vi "Refresh Target List.vi"(6 "Supported Devices":u32[](array[numeric]), 8 "error in (no error)":errorcluster, 9 "OwningVI Ref":refnum<vi>, 10 "UI Ref Cluster":T4, 11 "Target Info Cache":T1={"USBTargetList"={"TargetList"=[], "Value"=-1, "Target RT Info List"=[]}, "WiFiTargetList"={"TargetList"=[], "Value"=-1, "Target RT Info List"=[]}, "GenericTargetList"={"TargetList"=[], "Value"=-1, "Target RT Info List"=[]}, "IPTargetList"={"IP Error Out"={"status"=FALSE, "code"=0, "source"=""}, "Target RT Info List"=[]}} {"IPTargetList"."Target RT Info List"."ProdID" format="%.0x"; "USBTargetList"."Target RT Info List"."ProdID" format="%.0x"; "WiFiTargetList"."Target RT Info List"."ProdID" format="%.0x"; "GenericTargetList"."Target RT Info List"."ProdID" format="%.0x"}) -> (0 "error out":errorcluster, 3 "Target Info Cache Output":T1 {"IPTargetList"."Target RT Info List"."ProdID" format="%.0x"; "USBTargetList"."Target RT Info List"."ProdID" format="%.0x"; "WiFiTargetList"."Target RT Info List"."ProdID" format="%.0x"; "GenericTargetList"."Target RT Info List"."ProdID" format="%.0x"})   [LabVIEW 2021, in "myRIOMetaDataObj.lvclass"]
uses:
  myRIOMetaDataObj.lvclass
  WizardUIRef.ctl
  AvailableTargets.ctl
  TargetInfoHistory.ctl
  TargetListInfo.ctl
  <resource>/myRIO/Target Info.ctl
  InternalErrorCodes.vi
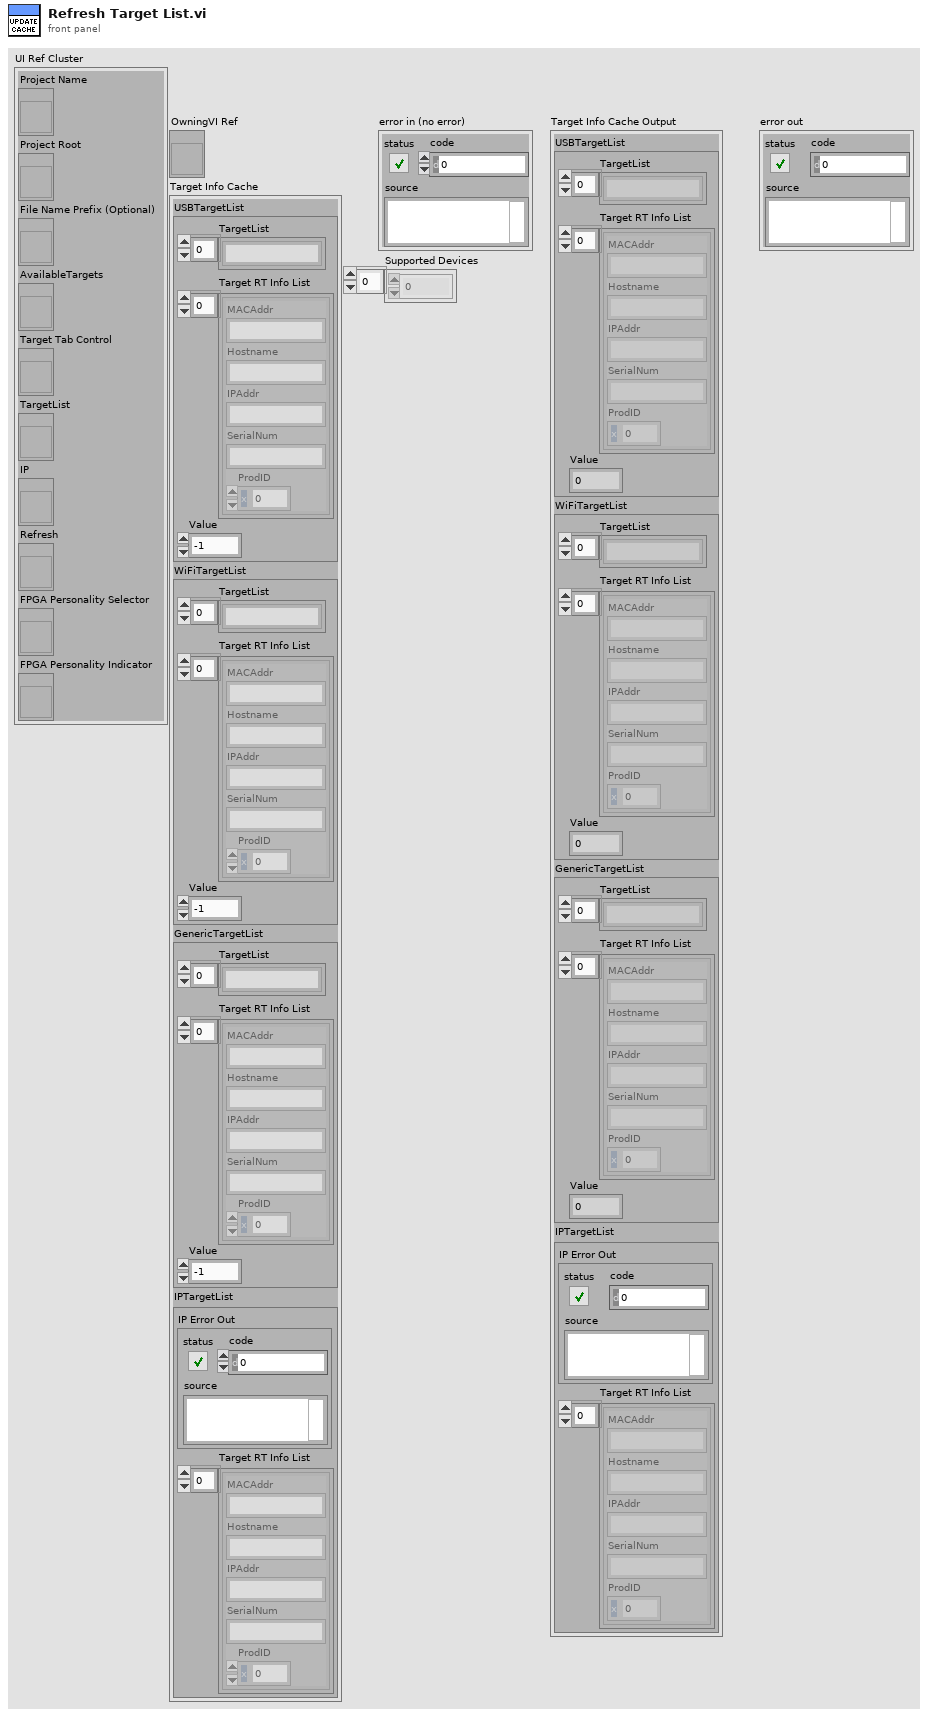
[diagram p1: front panel]
types:
  T1 = typedef "myRIOMetaDataObj.lvclass/TargetInfoHistory.ctl" = cluster{"USBTargetList":T2, "WiFiTargetList":T2, "GenericTargetList":T2, "IPTargetList":cluster{"IP Error Out":errorcluster, "Target RT Info List":T3[]}}
  T2 = typedef "myRIOMetaDataObj.lvclass/TargetListInfo.ctl" = cluster{"TargetList":string[], "Value":i32, "Target RT Info List":T3[]}
  T3 = typedef "Target Info.ctl" = cluster{"MACAddr":string, "Hostname":string, "IPAddr":string, "SerialNum":string, "ProdID":u32}
  T4 = typedef "myRIOMetaDataObj.lvclass/WizardUIRef.ctl" = cluster{"Project Name":refnum<vi>, "Project Root":refnum<vi>, "File Name Prefix (Optional)":refnum<vi>, "AvailableTargets":refnum<vi>, "Target Tab Control":refnum<vi>, "TargetList":refnum<vi>, "IP":refnum<vi>, "Refresh":refnum<vi>, "FPGA Personality Selector":refnum<vi>, "FPGA Personality Indicator":refnum<vi>}
  T5 = enum8{"Enabled", "Disabled", "Disabled and Grayed Out"}
  T6 = enum32{"USBTarget", "WifiTarget", "NoSpecificTarget", "TargetIP"}
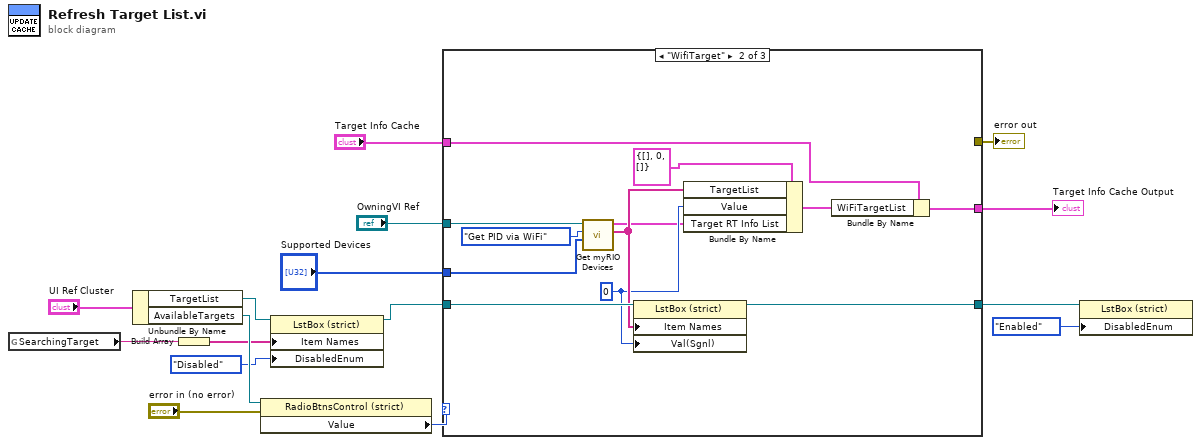
[diagram p0: block diagram]
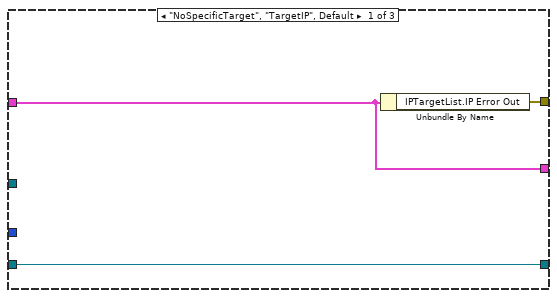
[diagram p2: hidden frame]
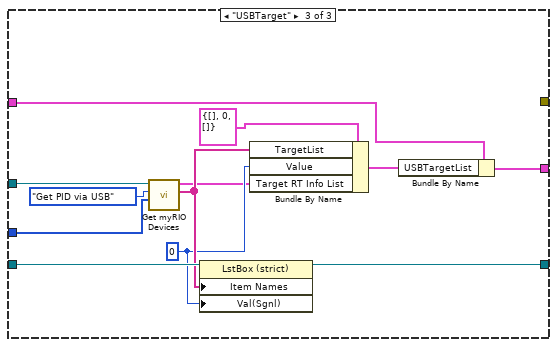
[diagram p3: hidden frame]
diagram:
  n1 = global read "InternalErrorCodes.vi" "SearchingTarget"() -> (w9:string)
  n2 = Unbundle By Name("UI Ref Cluster") -> ("TargetList"=w11:refnum<vi>, "AvailableTargets"=w15:refnum<vi>)
  n3 = Build Array(w9) -> (w8:string[])
  n4 = property class="RadioBtnsControl (strict)"(reference=w15, error in="error in (no error)") -> ("Value"=w6:T6)  [unwired: 2 out]
  n5 = property class="LstBox (strict)"(reference=w11, "Item Names"=w8, "DisabledEnum"=T5."Disabled" ("Disabled")) -> (reference out=w10:refnum<vi>)  [unwired: 1 in, 1 out]
  n6 = case shown="\"WifiTarget\"" w6 {
    tunnel: "OwningVI Ref" -> [_ w30 w42]
    tunnel: "Target Info Cache" -> [w18 w24 w36]
    tunnel: [w18 w23 w34] -> w14
    tunnel: [w19 _ _] -> w12
    tunnel: w10 -> [w17 w28 w40]
    tunnel: [w17 w21 w33] -> w3
    tunnel: "Supported Devices" -> [_ w20 w32]
    frame "NoSpecificTarget", "TargetIP", Default {
      n7 = Unbundle By Name(w18) -> ("IPTargetList.IP Error Out"=w19:errorcluster)
    }
    frame "WifiTarget" {
      w26 = 0 ("Value")
      n8 = call "Get myRIO Devices.vi"("Supported Devices"=w20, "Operation"=enum16{"Get PID via USB", "Get PID via WiFi"}."Get PID via WiFi", "OwningVI"=w30) -> ("TargetList"=w27:string[], "Detected Targets Info"=w25:T3[])  [unwired: 6 in, 1 out]
      n9 = property class="LstBox (strict)"(reference=w28, "Item Names"=w27, "Val(Sgnl)"=w26) -> (reference out=w21:refnum<vi>)  [unwired: 1 in, 1 out]
      n10 = Bundle By Name(cluster=T2 {"TargetList"=[], "Value"=0, "Target RT Info List"=[]} ("TargetListInfo"), "TargetList"=w27, "Value"=w26, "Target RT Info List"=w25) -> (w22:T2)
      n11 = Bundle By Name(cluster=w24, "WiFiTargetList"=w22) -> (w23:T1)
    }
    frame "USBTarget" {
      w38 = 0 ("Value")
      n12 = call "Get myRIO Devices.vi"("Supported Devices"=w32, "Operation"=enum16{"Get PID via USB", "Get PID via WiFi"}."Get PID via USB", "OwningVI"=w42) -> ("TargetList"=w39:string[], "Detected Targets Info"=w37:T3[])  [unwired: 6 in, 1 out]
      n13 = property class="LstBox (strict)"(reference=w40, "Item Names"=w39, "Val(Sgnl)"=w38) -> (reference out=w33:refnum<vi>)  [unwired: 1 in, 1 out]
      n14 = Bundle By Name(cluster=T2 {"TargetList"=[], "Value"=0, "Target RT Info List"=[]} ("TargetListInfo"), "TargetList"=w39, "Value"=w38, "Target RT Info List"=w37) -> (w35:T2)
      n15 = Bundle By Name(cluster=w36, "USBTargetList"=w35) -> (w34:T1)
    }
  }
  "Target Info Cache Output" <- w14
  "error out" <- w12
  n16 = property class="LstBox (strict)"(reference=w3, "DisabledEnum"=T5."Enabled" ("Disabled")) -> ()  [unwired: 1 in, 2 out]
